vi "Vec2TandData.vi"(11 "Frames":u32[](array[numeric])) -> (2 "_64Bits":u64, 3 "时间(秒)":dbl)   [LabVIEW 2015]
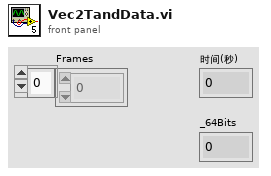
[diagram p1: front panel]
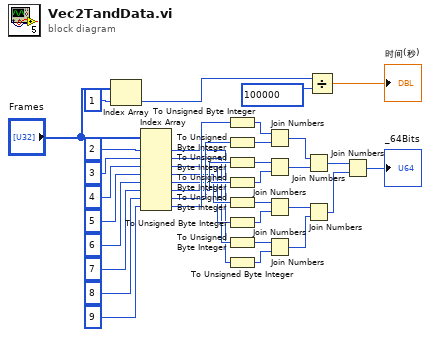
[diagram p0: block diagram]
diagram:
  n1 = Index Array(array="Frames", index=1 ("索引")) -> (element=w2:u32)
  n2 = Index Array(array="Frames", index #1=2 ("索引"), index #2=3 ("索引"), index #3=4 ("索引"), index #4=5 ("索引"), index #5=6 ("索引"), index #6=7 ("索引"), index #7=8 ("索引"), index #8=9 ("索引")) -> (element #1=w29:u32, element #2=w30:u32, element #3=w31:u32, element #4=w32:u32, element #5=w33:u32, element #6=w34:u32, element #7=w35:u32, element #8=w36:u32)
  n3 = To Unsigned Byte Integer(number=w36) -> (unsigned 8bit integer=w13:u8)
  n4 = To Unsigned Byte Integer(number=w35) -> (unsigned 8bit integer=w14:u8)
  n5 = To Unsigned Byte Integer(number=w34) -> (unsigned 8bit integer=w11:u8)
  n6 = To Unsigned Byte Integer(number=w33) -> (unsigned 8bit integer=w12:u8)
  n7 = To Unsigned Byte Integer(number=w32) -> (unsigned 8bit integer=w8:u8)
  n8 = To Unsigned Byte Integer(number=w31) -> (unsigned 8bit integer=w7:u8)
  n9 = To Unsigned Byte Integer(number=w30) -> (unsigned 8bit integer=w5:u8)
  n10 = To Unsigned Byte Integer(number=w29) -> (unsigned 8bit integer=w6:u8)
  n11 = Join Numbers(hi=w13, lo=w14) -> ((hi.lo)=w16:u16)
  n12 = Join Numbers(hi=w11, lo=w12) -> ((hi.lo)=w15:u16)
  n13 = Join Numbers(hi=w8, lo=w7) -> ((hi.lo)=w10:u16)
  n14 = Join Numbers(hi=w5, lo=w6) -> ((hi.lo)=w9:u16)
  n15 = Join Numbers(hi=w16, lo=w15) -> ((hi.lo)=w18:u32)
  n16 = Join Numbers(hi=w10, lo=w9) -> ((hi.lo)=w17:u32)
  n17 = Divide(x=w2, y=u32 100000) -> (x/y=→"时间(秒)":dbl)
  n18 = Join Numbers(hi=w18, lo=w17) -> ((hi.lo)=→"_64Bits":u64)
